vi "DigitalOscilloscope.vi"() -> ()   [LabVIEW 2014]
doc: "This is a VI made to be a digital oscilliscope. \nWe have measured a 1Hz input with a small number of samples (10), to test the voltage resolution formula given in the text. Our triangle wave was 10V pk-pk. In the scope, we see that the line is actually not a strait line, but is off set due to the voltage resolution of the DAQ. The scope shows it varies about 1mV. From the formula however, we expect to see 10V/2^16 ~ .15mV, so about 10 times less than what we observed. We checked the manual for our DAQ in the help files to determine our DAQ stores voltages with 16 bit values."
panel:
  out "Waveform Graph":dynamicdata(graph)=[{"t0"=timestamp(3496342833.0902863 s since 1904-01-01), "dt"=0.001, "Y"=[-5.0590029644279415, -5.054399318988087, -5.037300064318881, -5.023489127651193, -5.010335854465849, -4.992907767243666, -4.9813986528840735, -4.964628228881906, -4.952461450521127, -4.938321680903561], "attributes"=variant("NI_ChannelName"=variant(string "Voltage"), "NI_UnitDescription"=variant(string "Volts"))}]
  out "error out":errorcluster
  in  "Digitizing Parameters":T1={"Number of Samples"=10.0, "Sampling Frequency"=1000.0}
  in  "stop":bool
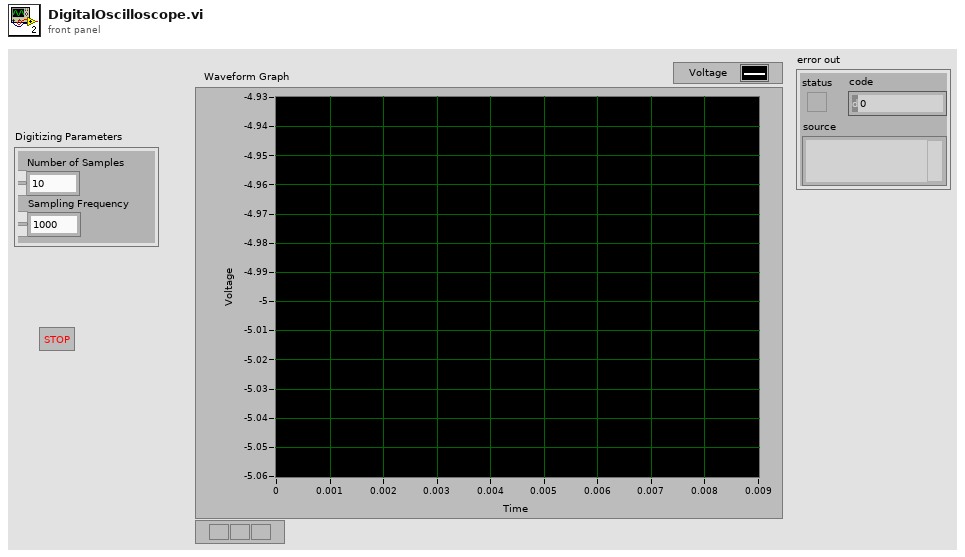
[diagram p1: front panel]
types:
  T1 = cluster{"Number of Samples":dbl, "Sampling Frequency":dbl}
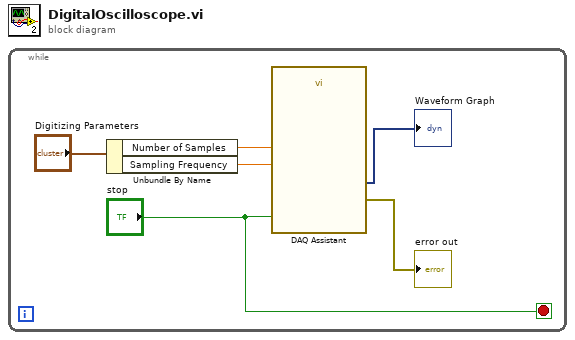
[diagram p0: block diagram]
diagram:
  n1 = while {
    stop <- "stop" stop-if-true
    n2 = Unbundle By Name("Digitizing Parameters") -> ("Number of Samples"=w5:dbl, "Sampling Frequency"=w4:dbl)
    n3 = call "DAQ Assistant"("rate"=w4, "number of samples"=w5, "stop (T)"="stop") -> ("data"=→"Waveform Graph":dynamicdata, "error out"=→"error out":errorcluster)  [unwired: 14 in, 1 out]
  }
